vi "Keithley 2220A 2230A 2231A Remote or Local.vi"(8 "error in (no error)":errorcluster, 10 "Go to Remote? (T: Yes)":bool=TRUE, 11 "VISA resource name":refnum<visa-resource-name>) -> (0 "error out":errorcluster, 3 "VISA resource name out":refnum<visa-resource-name>)   [LabVIEW 2019]
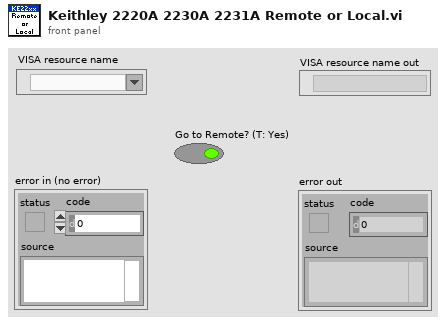
[diagram p1: front panel]
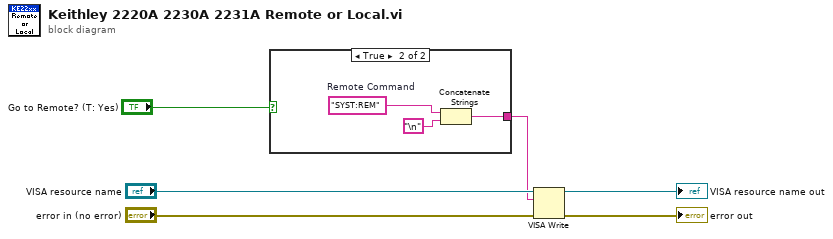
[diagram p0: block diagram]
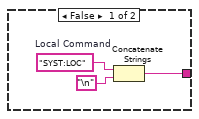
[diagram p2: hidden frame]
diagram:
  n1 = case shown="True" "Go to Remote? (T: Yes)" {
    tunnel: [w7 w10] -> w3
    frame False {
      w8 = "SYST:LOC"  # Local Command
      n2 = Concatenate Strings(w8, "\n") -> (w7:string)
    }
    frame True {
      w11 = "SYST:REM"  # Remote Command
      n3 = Concatenate Strings(w11, "\n") -> (w10:string)
    }
  }
  n4 = VISA Write(VISA resource name="VISA resource name", write buffer=w3, error in (no error)="error in (no error)") -> (VISA resource name out=→"VISA resource name out":refnum<visa-resource-name>, error out=→"error out":errorcluster)  [unwired: 1 out]
